vi "Main_Control_Panel.vi"() -> ()   [LabVIEW 2024]
panel:
  in  "Tab Control":enum32{"Manual Control", "Automaic Control"}(tab)
  in  "Kerosene Control Switch":bool
  in  "Purge Control Switch Channel":tag="Dev1/port0/line3"
  out "Purge Error":errorcluster
  in  "Code Stop":bool
  in  "GOX Control Switch":bool
  in  "GOX Control Switch Channel":tag="Dev1/port0/line1"
  out "GOX Error":errorcluster
  # "Torch Igniter Control Panel"
  # "Questions With Answers"
  # "How do the tab folders work?\n - Switch to the tab you wish to be in control of and press run to \ncammand the sub VIs to commence their sequence\n\nWhy is the manual control different?\n - The manual control is not a flat sequence sub VI, It is a while loop meaning that if you \nwant to do those controls run the code and then click the switch to activate the command\n\nCan I stop a sequence?\n  - Yes, you can stop them by pressing the stop button while the test is running.\n\n\nHow do the sub VIs work?\n - In every sub Vi there is another control pannel and code working. In our sub VIs there are flat sequences \n - that are structures that follow codes in set orders of operation. \n\nCan I change the timing of the Test tabs?\n - Yes, just change the times in the premade tabs."
  # "This tab is controlled by a while loop. \nPress the run command to activate the code, but \nto activate specific switches you must press the switches once the code is already running."
  # "This tab is not empty! It is connected to a sub VI. \nIf you want to start the process just stay on this tab \nand click \"run\" for the sequence to commence.\n\nThis sequence allows for opening two valves for a specified time.\n\nYou can stop the sequence by pressing the stop button which closes the two valves.\n\nIN CASE OF EMERGENCY  HIT PHYSCIAL STOP BUTTON\n(It will cut the power to the system)"
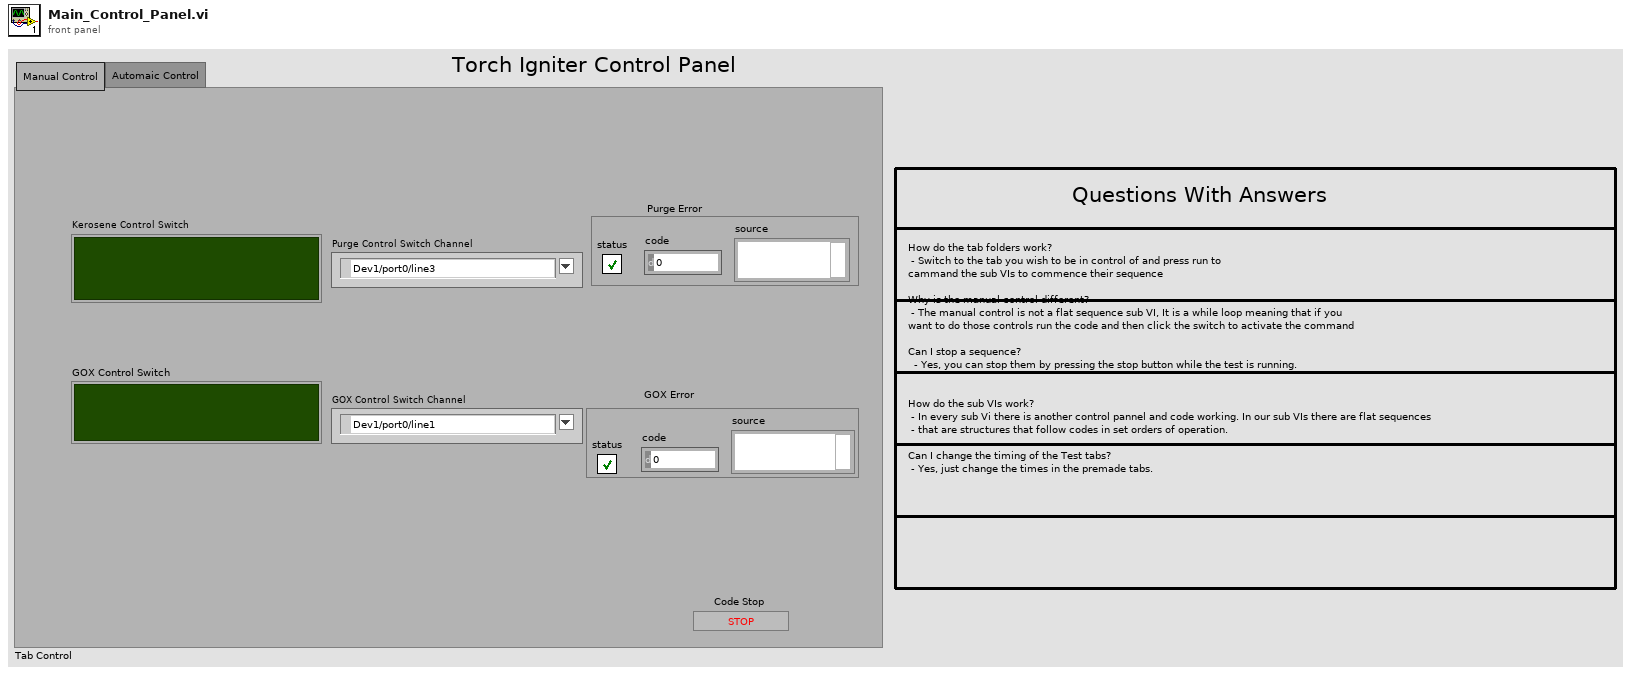
[diagram p1: front panel]
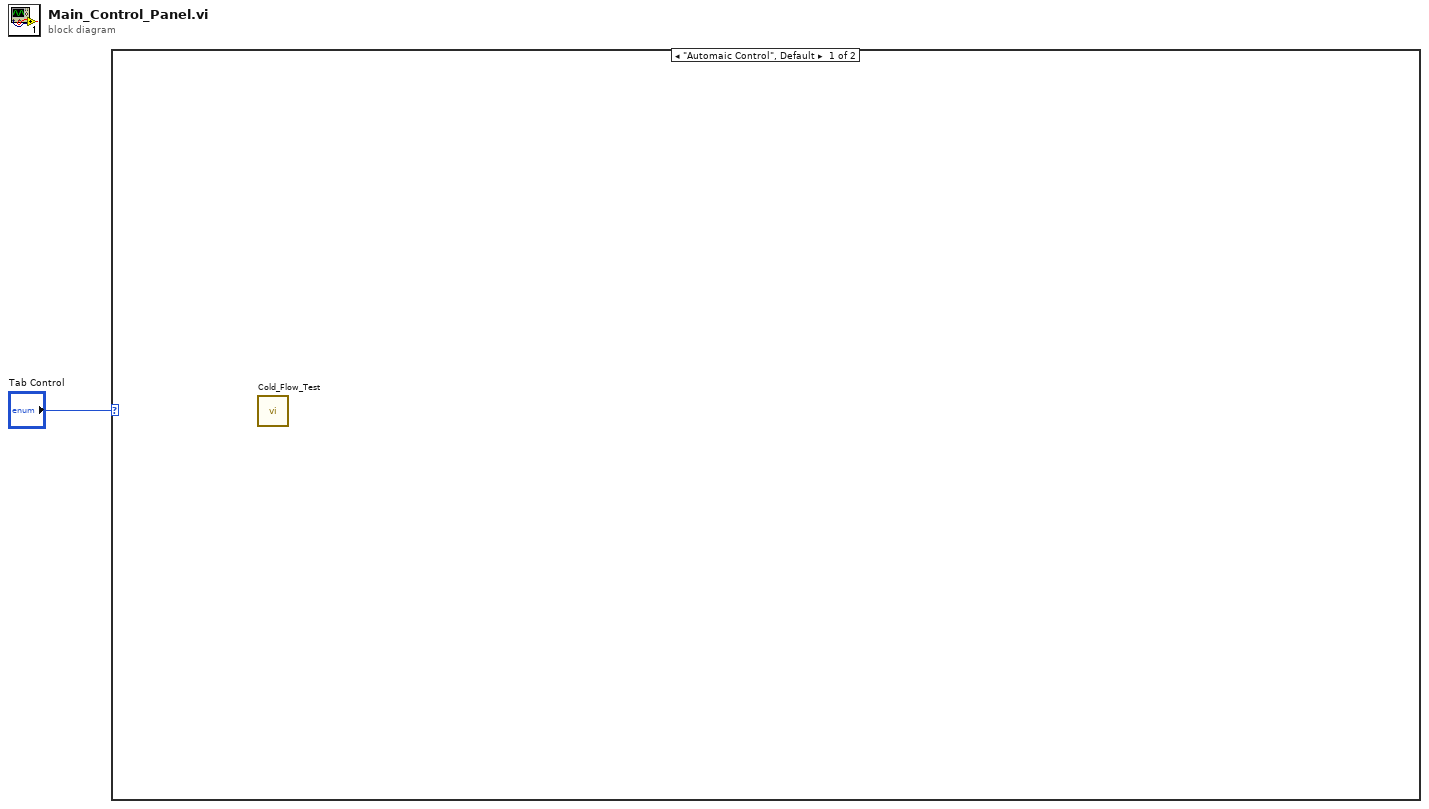
[diagram p0: block diagram]
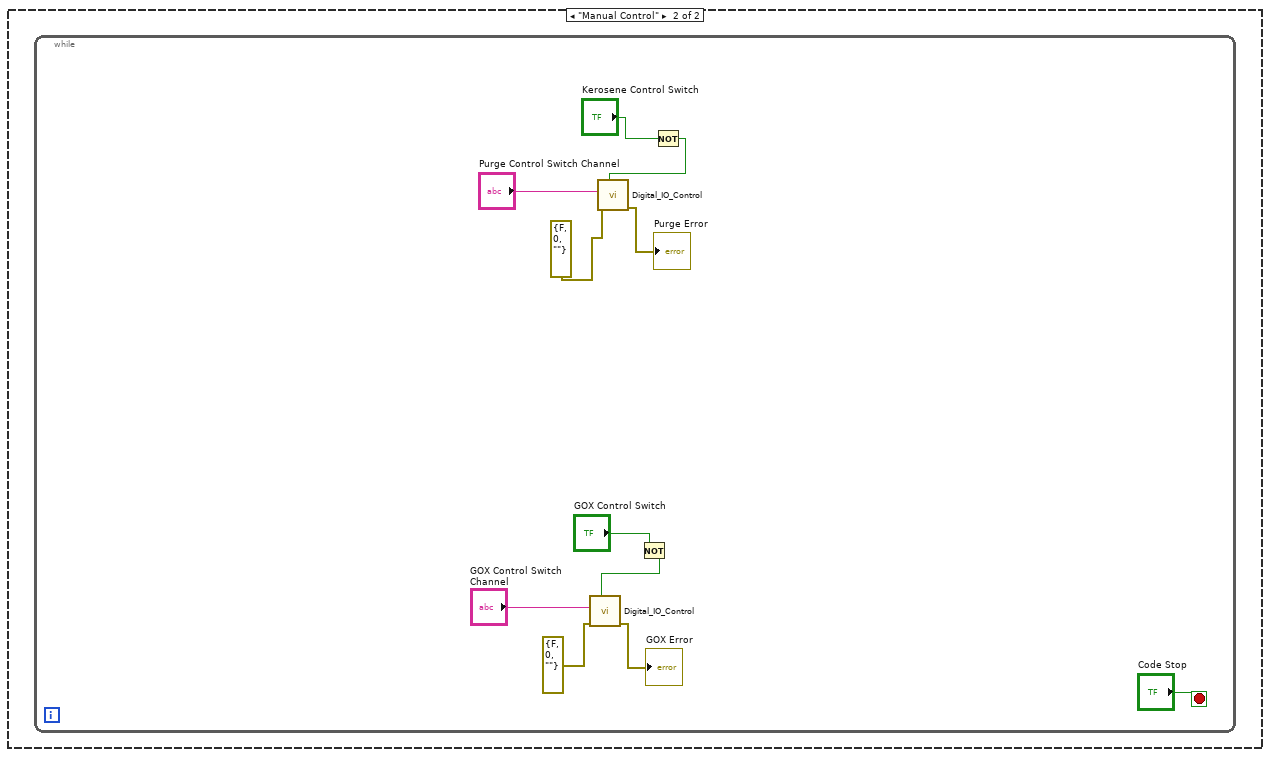
[diagram p2: hidden frame]
diagram:
  n1 = case shown="\"Automaic Control\", Default" "Tab Control" {
    frame "Automaic Control", Default {
      n2 = call "Cold_Flow_Test.vi"() -> ()  [unwired: 12 in]
    }
    frame "Manual Control" {
      n3 = while {
        stop <- "Code Stop" stop-if-true
        n4 = Not(x="GOX Control Switch") -> (.not. x?=w2:bool)
        n5 = call "Digital_IO_Control.vi"("Digital Channel High/Low (false : low)"=w2, "error in"=errorcluster {"status"=FALSE, "code"=0, "source"=""}, "Digital Port Seclection"="GOX Control Switch Channel") -> ("error out"=→"GOX Error":errorcluster)  [unwired: 5 in]
        n6 = Not(x="Kerosene Control Switch") -> (.not. x?=w7:bool)
        n7 = call "Digital_IO_Control.vi"("Digital Channel High/Low (false : low)"=w7, "error in"=errorcluster {"status"=FALSE, "code"=0, "source"=""}, "Digital Port Seclection"="Purge Control Switch Channel") -> ("error out"=→"Purge Error":errorcluster)  [unwired: 5 in]
      }
    }
  }
